vi "delete.vi"(8 "error in":errorcluster, 11 "type in":refnum<class "type.lvclass">) -> (0 "error out":errorcluster, 3 "type out":refnum<class "type.lvclass">)   [LabVIEW 2020, in "type.lvclass"]
uses:
  type.lvclass
  Nominal Client/Nominal Client.lvclass
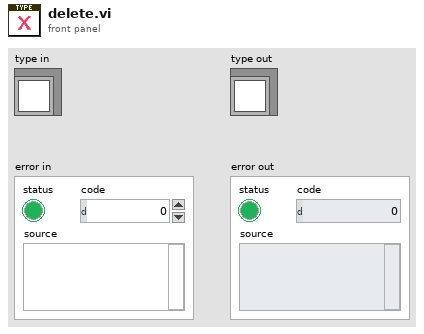
[diagram p1: front panel]
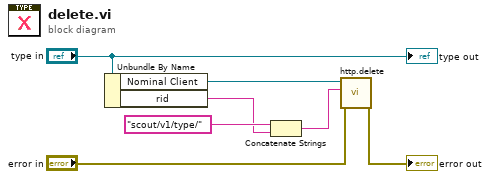
[diagram p0: block diagram]
diagram:
  n1 = Unbundle By Name("type in") -> ("Nominal Client"=w7:refnum<class "Nominal Client.lvclass">, "rid"=w5:string)
  n2 = Concatenate Strings("scout/v1/type/" ("Path"), w5) -> (w4:string)
  n3 = call "http.delete.vi"("error in"="error in", "Path"=w4, "Nominal Client in"=w7) -> ("error out"=→"error out":errorcluster)  [unwired: 6 in, 2 out]
  "type out" <- "type in"
